vi "Icai 105 - Simultry5.vi"() -> ()   [LabVIEW 2010]
uses:
  <vilib>/Utility/error.llb/DialogType.ctl
  <vilib>/DAQmx/write.llb/DAQmx Write (Analog DBL 1Chan 1Samp).vi
  <vilib>/DAQmx/write.llb/DAQmx Write (Analog 1D Wfm NChan NSamp).vi
  <vilib>/DAQmx/write.llb/DAQmx Write (Analog Wfm 1Chan NSamp).vi
  <vilib>/DAQmx/create/channels.llb/DAQmx Create Channel (AO-Voltage-Basic).vi
  <vilib>/daqmx/miscellaneous.llb/DAQmx Fill In Error Info.vi
  <vilib>/Waveform/WDTOps.llb/WDT Append Waveforms DBL.vi
  <vilib>/DAQmx/configure/timing.llb/DAQmx Timing (Sample Clock).vi
  <vilib>/measure/NI_MABase.lvlib
panel:
  in  "Rising Logic Output Chan":tag="Dev1/ao2"
  in  "Modulation Duration samples / 2":i32=150000
  out "Multiplier to arrive at Modulation # of samples":dbl=297.555285
  in  "Samples (1Ms/s)":i32=700000
  out "min value":dbl
  in  "Falling Logic Output Chan":tag="Dev1/ao1"
  in  "FM Waveform Channel":tag="Dev1/ao3"
  out "error out":errorcluster caption="error out (DAQ)"
  out "Mod":dbl=118572.0
  out "Numeric 2":dbl=3900000.0 format="%#_7g"
  out "Numeric":dbl=3900000.0 format="%#_7g"
  in  "CAI/ICAI":bool=TRUE
  in  "Pre-Trig Samples":ext=500.0 format="%.2f"
  out "?":dbl=579698.7113293351 format="%#_6f"
  in  "Fs":dbl=1000000.0
  out "#s":dbl=39524.02451426849
  in  "Time int":i32=30000
  in  "Sensitivity":u16(ring)=14 items=["2 nV/fA", "5 nV/fA", "10 nV/fA", "20 nV/fA", "50 nV/fA", "100 nV/fA", "200 nV/fA", "500 nV/fA", "1 uV/pA", "2 uV/pA", "5 uV/pA", "10 uV/pA", "20 uV/pA", "50 uV/pA", "100 uV/pA", "200 uV/pA", "500 uV/pA", "1 mV/nA", "2 mV/nA", "5 mV/nA", "10 mV/nA", "20 mV/nA", "50 mV/nA", "100 mV/nA", "200 mV/nA", "500 mV/nA", "1 V/uA"]
  in  "Detection Bandwidth":u16(ring)=7 items=["10 us/ 25 kHz", "30 us /8.33 kHz", "100 us/ 2.50 kHz", "300 us/ 833 Hz", "1 ms /250 Hz", "3 ms /83.3 Hz", "10 ms/ 25 Hz", "30 ms/ 8.33 Hz", "100 ms/ 2.50 Hz", "300 ms/ 0.833 Hz ", "1 s/ 0.250 Hz", "3 s/ 0.0833 Hz", "10 s/0.025 Hz"]
  in  "SR 830 GPIB Address":i32=8
  in  "Freq 2":dbl=2490.2 format="%_7g"
  out "Iterat #":dbl=10.0
  in  "Iteration":dbl=17.0
  in  "stop 2":bool
  in  "pulse":bool=TRUE
  in  "Start":ext=0.05
  out "?":waveform(dbl)[](graph)
  in  "amplitude 2":dbl=0.2 format="%0.2p"
  in  "?":T1(ring)
  in  "phase 2":dbl format="%.2p"
  in  "Offset 2":dbl=-0.0 format="%#_6p"
  in  "frequency 4":dbl=100.0 format="%0.2p"
  in  "sampling info 4":cluster{"Fs":dbl, "#s":dbl}={"Fs"=1000000.0, "#s"=2500.0} {"Fs" format="%.2p"}
  in  "?":T1(ring)=enum."Triangle Wave"
  in  "offset 4":dbl=-1.0 format="%0.2p"
  in  "phase 4":dbl=90.0 format="%.2p"
  in  "amplitude 4":dbl=1.0 format="%0.2p"
  in  "frequency 1":dbl=100.0 format="%0.2p"
  in  "amplitude 1":dbl=1.0 format="%0.2p"
  in  "sampling info 1":cluster{"Fs":dbl, "#s":dbl}={"Fs"=1000000.0, "#s"=2500.0} {"Fs" format="%.2p"}
  in  "?":T1(ring)=enum."Triangle Wave"
  in  "phase 1":dbl=-90.0 format="%.2p"
  in  "Offset 1":dbl format="%#_6p"
  in  "iterat":dbl=1.0
  out "CW":dbl=123571.0
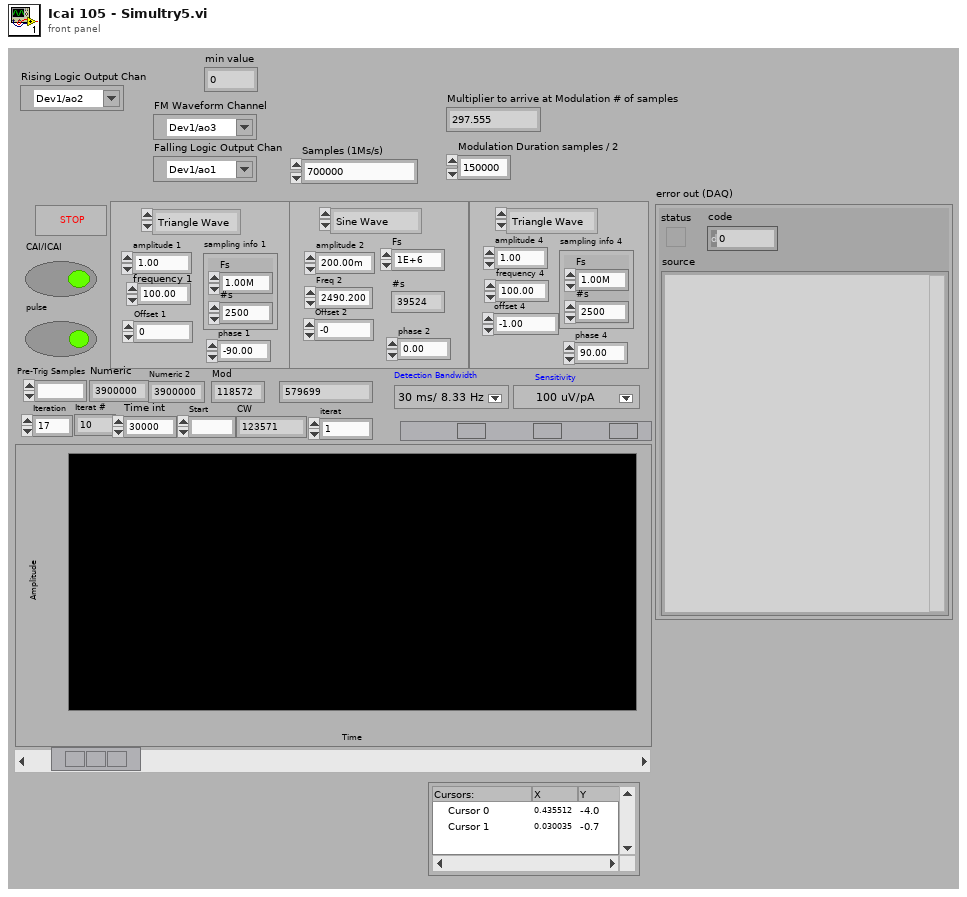
[diagram p1: front panel]
types:
  T1 = enum16{"Sine Wave", "Triangle Wave", "Square Wave", "Sawtooth Wave"}
  T2 = typedef "DialogType.ctl" = u16
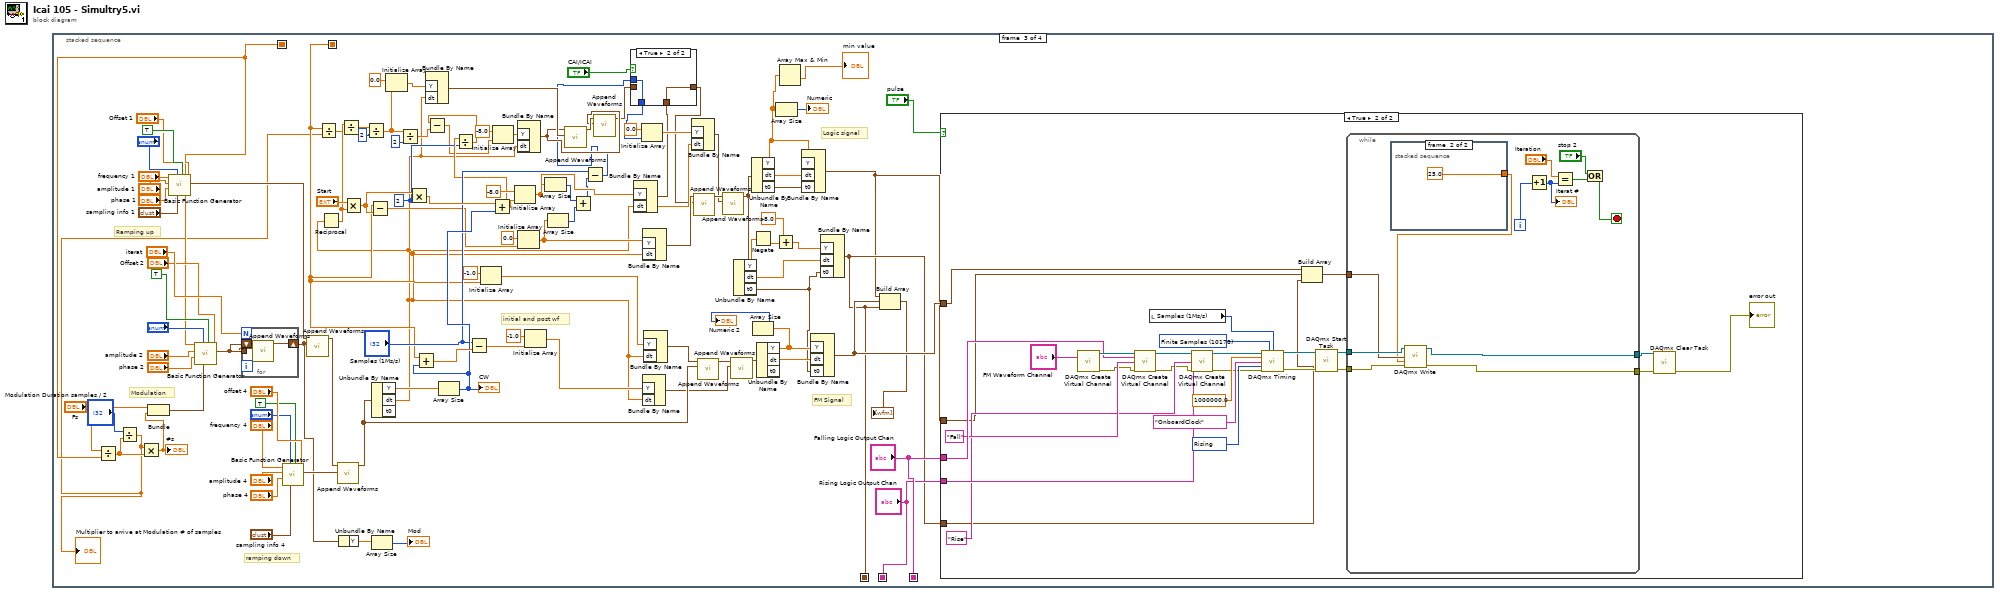
[diagram p0: block diagram]
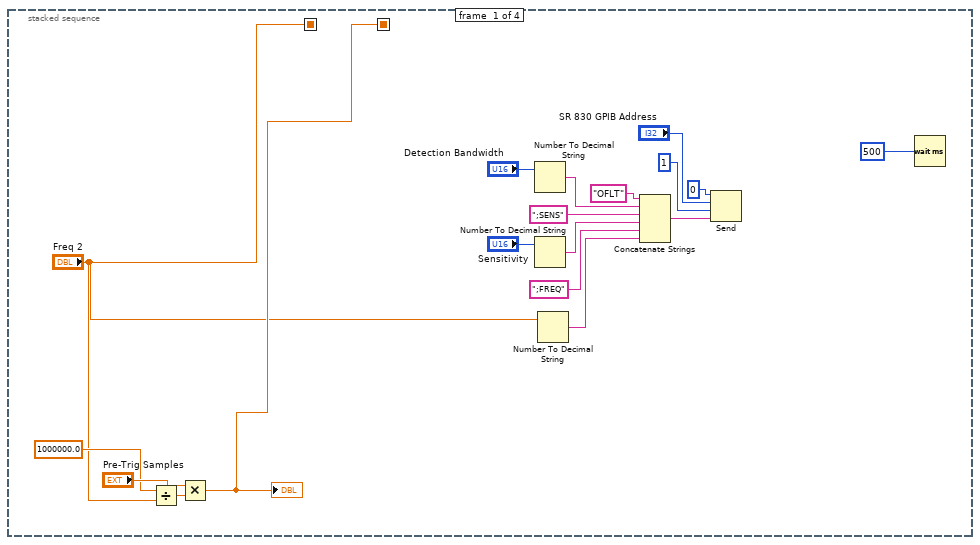
[diagram p2: hidden frame]
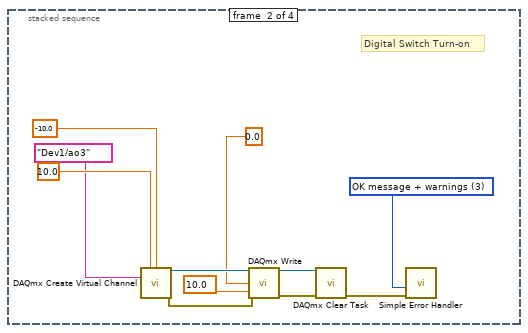
[diagram p3: hidden frame]
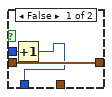
[diagram p4: hidden frame]
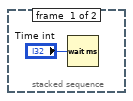
[diagram p6: hidden frame]
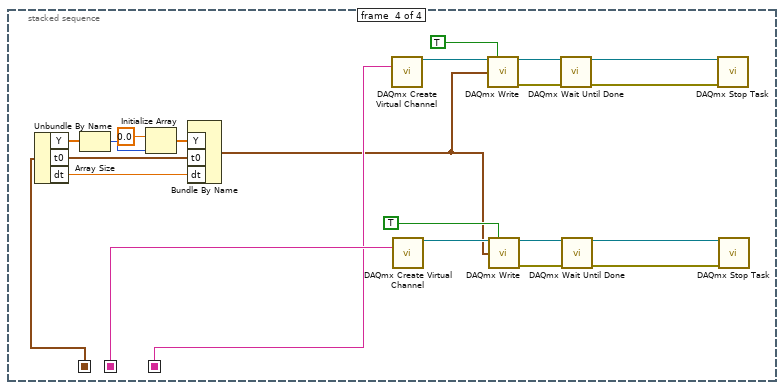
[diagram p7: hidden frame]
diagram:
  n1 = stacked-sequence {
    seq-local: ["Freq 2" _ _ _] -> [_ _ w84 _]
    seq-local: [w4 _ _ _] -> [_ _ w71 _]
    seq-local: [_ _ "Falling Logic Output Chan" _] -> [_ _ _ w192]
    seq-local: [_ _ "Rising Logic Output Chan" _] -> [_ _ _ w193]
    seq-local: [_ _ w32 _] -> [_ _ _ w207]
    frame #0 {
      n2 = Divide(x=1000000.0 ("Fs 2"), y="Freq 2") -> (x/y=w7:dbl)
      n3 = Multiply(x="Pre-Trig Samples", y=w7) -> (x*y=w4:ext)
      "?" <- w4
      n4 = Number To Decimal String(number="Detection Bandwidth") -> (decimal integer string=w17:string)  [unwired: 1 out]
      n5 = Number To Decimal String(number="Sensitivity") -> (decimal integer string=w15:string)  [unwired: 1 out]
      n6 = Number To Decimal String(number="Freq 2") -> (decimal integer string=w2:string)  [unwired: 1 out]
      n7 = Concatenate Strings("OFLT", w17, ";SENS", w15, ";FREQ" ("string"), w2) -> (w14:string)
      n8 = Send(0:0 ("bus"), 2:"SR 830 GPIB Address", 3:i16 1 ("mode"), 5:w14) -> ()  [unwired: 1 in, 3 out]
      n9 = Wait (ms)(milliseconds to wait=500) -> ()  [unwired: 1 out]
    }
    frame #1 {
      w22 = T2 3 items=["no dialog", "OK message", "continue or stop message", "OK message + warnings", "continue/stop + warnings"] ("type of dialog (OK msg:1)")
      # "Digital Switch Turn-on"
      n10 = call-poly <vilib>:"DAQmx Create Virtual Channel.vi"("maximum value"=10.0 ("Maximum Value"), "minimum value"=-10.0 ("Minimum Value"), "physical channels"=tag "Dev1/ao3" ("Physical Channel")) -> ("task out"=w25:refnum<k21>, "error out"=w26:errorcluster)  [unwired: 6 in, 5 out]
      n11 = call-poly <vilib>:"DAQmx Write.vi"("task/channels in"=w25, "data"=0.0 ("Voltage Output"), "timeout"=10.0, "error in"=w26) -> ("task out"=w20:refnum<k21>, "error out"=w21:errorcluster)  [unwired: 1 in, 9 out]
      n12 = call <vilib>:"DAQmx Clear Task.vi"("task in"=w20, "error in"=w21) -> ("error out"=w19:errorcluster)  [unwired: 13 out]
      n13 = call <vilib>:"Simple Error Handler.vi"("type of dialog (OK msg:1)"=w22, "error in (no error)"=w19) -> ()  [unwired: 8 out]
    }
    frame #2 {
      w79 = 2
      # "initial and post wf"
      # "FM Signal"
      # "Logic signal"
      # "Ramping up"
      # "ramping down"
      # "Modulation"
      n14 = Divide(x="Fs", y=w84) -> (x/y=w45:dbl)
      n15 = Divide(x="Modulation Duration samples / 2", y=w45) -> (x/y=w44:dbl)
      "Multiplier to arrive at Modulation # of samples" <- w44
      n16 = Multiply(x=w44, y=w45) -> (x*y=w47:dbl)
      "#s" <- w47
      n17 = Bundle("Fs"="Fs", w47) -> (w82:cluster{"Fs":dbl, dbl})  [unwired: 1 out]
      n18 = call <vilib>:"Basic Function Generator.vi"("offset"="Offset 1", "reset signal"=TRUE, "sampling info"="sampling info 1", "signal type"="?", "phase"="phase 1", "amplitude"="amplitude 1", "frequency"="frequency 1") -> ("signal out"=w120:waveform(dbl))  [unwired: 2 in, 2 out]
      n19 = call <vilib>:"Basic Function Generator.vi"("offset"="Offset 2", "reset signal"=TRUE, "sampling info"=w82, "signal type"="?", "phase"="phase 2", "amplitude"="amplitude 2", "frequency"=w84) -> ("signal out"=w85:waveform(dbl))  [unwired: 2 in, 2 out]
      n20 = for {
        N: "iterat" -> [_]
        shift-right: [w190] -> w50
        shift-left: w85 -> [w188]
        tunnel: w85 -> [w189]
        n21 = call-poly <vilib>:"Append Waveforms.vi"("waveform B"=w189, "waveform A"=w188) -> ("waveform out"=w190:waveform(dbl))  [unwired: 1 in, 8 out]
      }
      n22 = call <vilib>:"Basic Function Generator.vi"("offset"="offset 4", "reset signal"=TRUE, "sampling info"="sampling info 4", "signal type"="?", "phase"="phase 4", "amplitude"="amplitude 4", "frequency"="frequency 4") -> ("signal out"=w125:waveform(dbl))  [unwired: 2 in, 2 out]
      n23 = call-poly <vilib>:"Append Waveforms.vi"("waveform B"=w50, "waveform A"=w120) -> ("waveform out"=w119:waveform(dbl))  [unwired: 1 in, 8 out]
      n24 = Divide(x=w71, y=w44) -> (x/y=w72:ext)
      n25 = call-poly <vilib>:"Append Waveforms.vi"("waveform B"=w125, "waveform A"=w119) -> ("waveform out"=w118:waveform(dbl))  [unwired: 1 in, 8 out]
      n26 = Unbundle By Name(w50) -> ("Y"=w51:dbl[])
      n27 = Array Size(array=w51) -> (size(s)=→"Mod":i32)
      n28 = Unbundle By Name(w118) -> ("Y"=w121:dbl[], "dt"=w63:dbl)  [unwired: 1 out]
      n29 = Reciprocal(x=w63) -> (1/x=w73:dbl)
      n30 = Divide(x=w73, y=w72) -> (x/y=w69:ext)
      n31 = Multiply(x="Start", y=w73) -> (x*y=w95:ext)
      n32 = Divide(x=w69, y=2) -> (x/y=w66:ext)
      n33 = Subtract(x=w71, y=w95) -> (x-y=w96:ext)
      n34 = Initialize Array(0.0 ("Trigger down"), w66) -> (w76:dbl[])
      n35 = Divide(x=w66, y=2) -> (x/y=w64:ext)
      n36 = Multiply(x=w95, y=w79) -> (x*y=w103:ext)
      n37 = Bundle By Name("Y"=w76, "dt"=w63) -> (w75:waveform(dbl))  [unwired: 1 out]
      n38 = Array Size(array=w121) -> (size(s)=w102:i32)
      "CW" <- w102
      n39 = Add(x=w71, y=w102) -> (x+y=w107:ext)
      n40 = Subtract(x="Samples (1Ms/s)", y=w107) -> (x-y=w106:ext)
      n41 = Initialize Array(-1.0 ("DC level"), w71) -> (w109:dbl[])
      n42 = Add(x=w103, y=w102) -> (x+y=w80:ext)
      n43 = Divide(x=w80, y=w79) -> (x/y=w68:ext)
      n44 = Subtract(x=w68, y=w64) -> (x-y=w67:ext)
      n45 = Initialize Array(-8.0 ("Trigger up"), w67) -> (w78:dbl[])
      n46 = Initialize Array(-8.0 ("Trigger up"), w80) -> (w93:dbl[])
      n47 = Bundle By Name("Y"=w78, "dt"=w63) -> (w62:waveform(dbl))  [unwired: 1 out]
      n48 = Initialize Array(0.0 ("Trigger down"), w96) -> (w94:dbl[])
      n49 = Initialize Array(-1.0 ("DC level"), w106) -> (w105:dbl[])
      n50 = Array Size(array=w93) -> (size(s)=w91:i32)
      n51 = Array Size(array=w94) -> (size(s)=w92:i32)
      n52 = call-poly <vilib>:"Append Waveforms.vi"("waveform B"=w75, "waveform A"=w62) -> ("waveform out"=w74:waveform(dbl))  [unwired: 1 in, 8 out]
      n53 = Add(x=w91, y=w92) -> (x+y=w90:i32)
      n54 = Subtract(x="Samples (1Ms/s)", y=w90) -> (x-y=w54:i32)
      n55 = call-poly <vilib>:"Append Waveforms.vi"("waveform B"=w62, "waveform A"=w74) -> ("waveform out"=w61:waveform(dbl))  [unwired: 1 in, 8 out]
      n56 = Bundle By Name("Y"=w93, "dt"=w63) -> (w59:waveform(dbl))  [unwired: 1 out]
      n57 = case shown="True" "CAI/ICAI" {
        tunnel: w61 -> [w144 _]
        tunnel: [w144 w146] -> w60
        tunnel: w59 -> [_ w146]
        tunnel: w54 -> [w143 w145]
        tunnel: [w142 w145] -> w53
        frame False {
          n58 = Increment(x=w143) -> (x+1=w142:i32)
        }
        frame True {
        }
      }
      n59 = Initialize Array(0.0 ("Trigger down"), w53) -> (w99:dbl[])
      n60 = Bundle By Name("Y"=w105, "dt"=w63) -> (w104:waveform(dbl))  [unwired: 1 out]
      n61 = Bundle By Name("Y"=w94, "dt"=w63) -> (w98:waveform(dbl))  [unwired: 1 out]
      n62 = Bundle By Name("Y"=w109, "dt"=w63) -> (w123:waveform(dbl))  [unwired: 1 out]
      n63 = Bundle By Name("Y"=w99, "dt"=w63) -> (w97:waveform(dbl))  [unwired: 1 out]
      n64 = call-poly <vilib>:"Append Waveforms.vi"("waveform B"=w60, "waveform A"=w98) -> ("waveform out"=w115:waveform(dbl))  [unwired: 1 in, 8 out]
      n65 = call-poly <vilib>:"Append Waveforms.vi"("waveform B"=w118, "waveform A"=w123) -> ("waveform out"=w124:waveform(dbl))  [unwired: 1 in, 8 out]
      n66 = call-poly <vilib>:"Append Waveforms.vi"("waveform B"=w97, "waveform A"=w115) -> ("waveform out"=w43:waveform(dbl))  [unwired: 1 in, 8 out]
      n67 = call-poly <vilib>:"Append Waveforms.vi"("waveform B"=w104, "waveform A"=w124) -> ("waveform out"=w112:waveform(dbl))  [unwired: 1 in, 8 out]
      n68 = Unbundle By Name(w43) -> ("Y"=w42:dbl[], "dt"=w37:dbl, "t0"=w38:timestamp)
      n69 = Unbundle By Name(w43) -> ("Y"=w49:dbl[], "dt"=w113:dbl, "t0"=w39:timestamp)
      n70 = Negate(x=w42) -> (-x=w40:dbl[])
      n71 = Unbundle By Name(w112) -> ("Y"=w55:dbl[], "dt"=w111:dbl)  [unwired: 1 out]
      n72 = Array Size(array=w55) -> (size(s)=→"Numeric 2":i32)
      n73 = Add(x=-8.0, y=w40) -> (x+y=w36:dbl[])
      n74 = Array Size(array=w49) -> (size(s)=→"Numeric":i32)
      n75 = Array Max & Min(array=w49) -> (min value=→"min value":dbl)  [unwired: 3 out]
      n76 = Bundle By Name("Y"=w49, "dt"=w113, "t0"=w39) -> (w31:waveform(dbl))  [unwired: 1 out]
      n77 = Bundle By Name("Y"=w55, "dt"=w111, "t0"=w38) -> (w48:waveform(dbl))  [unwired: 1 out]
      n78 = Bundle By Name("Y"=w36, "dt"=w37, "t0"=w38) -> (w32:waveform(dbl))  [unwired: 1 out]
      n79 = Build Array(w31, w48, w32) -> (→"?":waveform(dbl)[])
      n80 = case shown="True" "pulse" {
        tunnel: w48 -> [_ w154]
        tunnel: w31 -> [_ w153]
        tunnel: w32 -> [_ w152]
        tunnel: "Falling Logic Output Chan" -> [_ w171]
        tunnel: "Rising Logic Output Chan" -> [_ w168]
        frame False {
        }
        frame True {
          w162 = 10178 items=["Finite Samples"=10178, "Continuous Samples"=10123, "Hardware Timed Single Point"=12522] ("sample mode")
          w164 = 10280 items=["Rising"=10280, "Falling"=10171] ("active edge")
          n81 = call-poly <vilib>:"DAQmx Create Virtual Channel.vi"("physical channels"="FM Waveform Channel") -> ("task out"=w172:refnum<k21>, "error out"=w156:errorcluster)  [unwired: 13 in]
          n82 = call-poly <vilib>:"DAQmx Create Virtual Channel.vi"("task in"=w172, "physical channels"=w171, "name to assign"="Fall", "error in"=w156) -> ("task out"=w169:refnum<k21>, "error out"=w157:errorcluster)  [unwired: 10 in]
          n83 = local read "Samples (1Ms/s)"() -> (w161:i32)
          n84 = call-poly <vilib>:"DAQmx Create Virtual Channel.vi"("task in"=w169, "physical channels"=w168, "name to assign"="Rise", "error in"=w157) -> ("task out"=w166:refnum<k21>, "error out"=w158:errorcluster)  [unwired: 10 in]
          n85 = call-poly <vilib>:"DAQmx Timing.vi"("task/channels in"=w166, "sample mode"=w162, "samples per channel"=w161, "rate"=1000000.0, "source"=tag "OnboardClock", "active edge"=w164, "error in"=w158) -> ("task out"=w160:refnum<k21>, "error out"=w159:errorcluster)  [unwired: 7 in]
          n86 = Build Array(w154, w153, w152) -> (w151:waveform(dbl)[])
          n87 = call <vilib>:"DAQmx Start Task.vi"("task/channels in"=w160, "error in"=w159) -> ("task out"=w155:refnum<k21>, "error out"=w150:errorcluster)  [unwired: 12 in]
          n88 = while {
            tunnel: w155 -> [w179]
            tunnel: w151 -> [w178]
            tunnel: w150 -> [w177]
            tunnel: [w176] -> w147
            tunnel: [w175] -> w149
            i -> [w182]
            stop <- w183 stop-if-true
            n89 = stacked-sequence {
              tunnel: [_ 25.0 ("timeout (s)")] -> w174
              frame #0 {
                n90 = Wait (ms)(milliseconds to wait="Time int") -> ()  [unwired: 1 out]
              }
              frame #1 {
              }
            }
            n91 = call-poly <vilib>:"DAQmx Write.vi"("task/channels in"=w179, "data"=w178, "timeout"=w174, "error in"=w177) -> ("task out"=w176:refnum<k21>, "error out"=w175:errorcluster)  [unwired: 9 in, 1 out]
            n92 = Increment(x=w182) -> (x+1=w180:i32)
            "Iterat #" <- w180
            n93 = Equal?(x="Iteration", y=w180) -> (x = y?=w185:bool)
            n94 = Or(x="stop 2", y=w185) -> (x .or. y?=w183:bool)
          }
          n95 = call <vilib>:"DAQmx Clear Task.vi"("task in"=w147, "error in"=w149) -> ("error out"=→"error out":errorcluster)  [unwired: 13 in]
        }
      }
    }
    frame #3 {
      n96 = Unbundle By Name(w207) -> ("Y"=w204:dbl[], "t0"=w206:timestamp, "dt"=w205:dbl)
      n97 = Array Size(array=w204) -> (size(s)=w203:i32)
      n98 = Initialize Array(0.0 ("element"), w203) -> (w201:dbl[])
      n99 = Bundle By Name("Y"=w201, "t0"=w206, "dt"=w205) -> (w191:waveform(dbl))  [unwired: 1 in]
      n100 = call-poly <vilib>:"DAQmx Create Virtual Channel.vi"("physical channels"=w192) -> ("task out"=w200:refnum<k21>)  [unwired: 13 in, 1 out]
      n101 = call-poly <vilib>:"DAQmx Create Virtual Channel.vi"("physical channels"=w193) -> ("task out"=w194:refnum<k21>)  [unwired: 13 in, 1 out]
      n102 = call-poly <vilib>:"DAQmx Write.vi"("task/channels in"=w200, "auto start"=TRUE, "data"=w191) -> ("task out"=w208:refnum<k21>, "error out"=w211:errorcluster)  [unwired: 10 in, 1 out]
      n103 = call-poly <vilib>:"DAQmx Write.vi"("task/channels in"=w194, "auto start"=TRUE, "data"=w191) -> ("task out"=w195:refnum<k21>, "error out"=w198:errorcluster)  [unwired: 10 in, 1 out]
      n104 = call <vilib>:"DAQmx Wait Until Done.vi"("task/channels in"=w208, "error in"=w211) -> ("task out"=w210:refnum<k21>, "error out"=w212:errorcluster)  [unwired: 12 in]
      n105 = call <vilib>:"DAQmx Wait Until Done.vi"("task/channels in"=w195, "error in"=w198) -> ("task out"=w197:refnum<k21>, "error out"=w199:errorcluster)  [unwired: 12 in]
      n106 = call <vilib>:"DAQmx Stop Task.vi"("task/channels in"=w210, "error in"=w212) -> ()  [unwired: 12 in, 2 out]
      n107 = call <vilib>:"DAQmx Stop Task.vi"("task/channels in"=w197, "error in"=w199) -> ()  [unwired: 12 in, 2 out]
    }
  }
